vi "smiley.vi"(10 "std threshold":dbl=-35.3, 11 "damp":dbl[](array[numeric])) -> (3 "Array":picture[](array[picture]))   [LabVIEW 2017]
panel:
  out "appended path":path
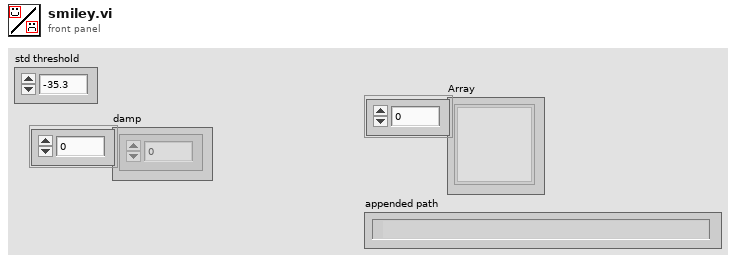
[diagram p1: front panel]
types:
  T1 = typedef "imagedata.ctl" = cluster{"image type":i32, "image depth":i32, "image":u8[], "mask":u8[], "colors":u32[], "Rectangle":cluster{"left":i16, "top":i16, "right":i16, "bottom":i16}}
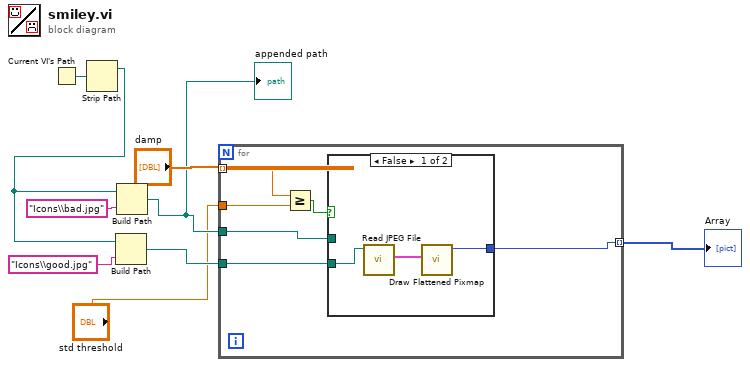
[diagram p0: block diagram]
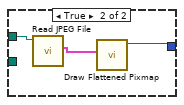
[diagram p2: hidden frame]
diagram:
  n1 = Current VI's Path() -> (path=w3:path)
  n2 = Strip Path(path=w3) -> (stripped path=w2:path)  [unwired: 1 out]
  n3 = Build Path(base path=w2, name or relative path="Icons\\good.jpg") -> (appended path=w5:path)
  n4 = Build Path(base path=w2, name or relative path="Icons\\bad.jpg") -> (appended path=w4:path)
  "appended path" <- w4
  n5 = for {
    tunnel: "damp" -> [w15] mode=indexing
    tunnel: w4 -> [w13]
    tunnel: w5 -> [w12]
    tunnel: [w11] -> w8 mode=indexing
    tunnel: "std threshold" -> [w10]
    n6 = Greater Or Equal?(x=w15, y=w10) -> (x >= y?=w14:bool)
    n7 = case shown="False" w14 {
      tunnel: w13 -> [_ w21]
      tunnel: w12 -> [w18 _]
      tunnel: [w16 w19] -> w11
      frame False {
        n8 = call <vilib>:"Read JPEG File.vi"("path to JPEG file"=w18) -> ("image data"=w17:T1)  [unwired: 8 in, 2 out]
        n9 = call <vilib>:"Draw Flattened Pixmap.vi"("image data"=w17) -> ("new picture"=w16:picture)  [unwired: 1 in, 7 out]
      }
      frame True {
        n10 = call <vilib>:"Read JPEG File.vi"("path to JPEG file"=w21) -> ("image data"=w20:T1)  [unwired: 8 in, 2 out]
        n11 = call <vilib>:"Draw Flattened Pixmap.vi"("image data"=w20) -> ("new picture"=w19:picture)  [unwired: 1 in, 7 out]
      }
    }
  }
  "Array" <- w8
